vi "deserialize (HW-Ballard).vi"(11 "data in":string[][](array[string])) -> (3 "hw configuration":T1[](array[typedef]))   [LabVIEW 2020]
uses:
  _controls/ballard1553_hw_map.ctl
  _controls/ballard1553_RT_list.ctl
  <vilib>/Utility/miscctls.llb/LVMapReplaceAction.ctl
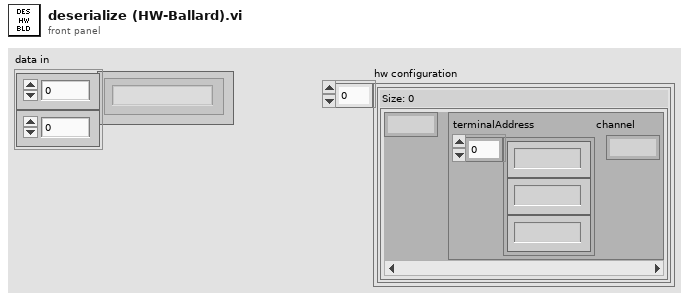
[diagram p1: front panel]
types:
  T1 = typedef "ballard1553_hw_map.ctl" = map{i32, T2}
  T2 = typedef "ballard1553_RT_list.ctl" = cluster{"terminalAddress":i32[], "channel":i32}
  T3 = typedef "LVMapReplaceAction.ctl" = enum32{"Modify Entry only if found", "Add or Modify Entry", "Delete Entry"}
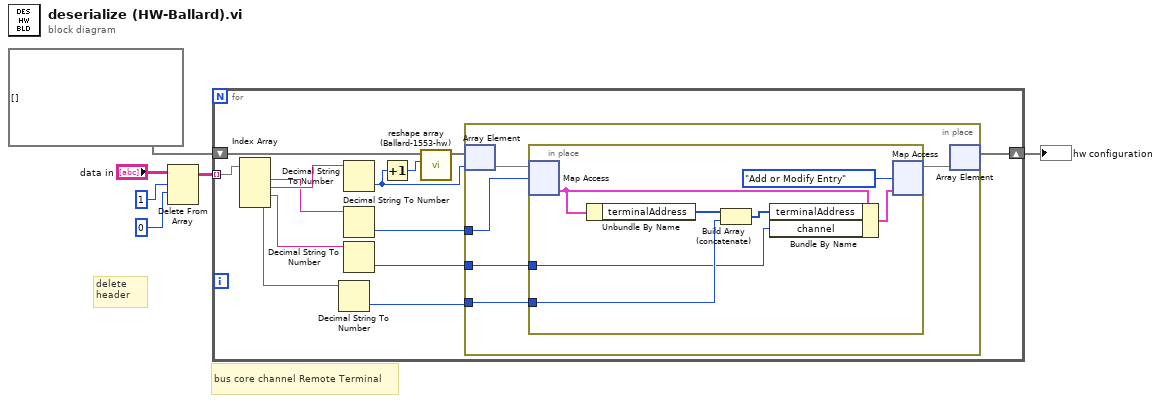
[diagram p0: block diagram]
diagram:
  # "bus\tcore\tchannel\tRemote Terminal"
  # "delete\nheader"
  n1 = Delete From Array(array="data in", length=1, index (row)=0) -> (array with subset deleted=w3:string[][])  [unwired: 1 in, 1 out]
  n2 = for {
    tunnel: w3 -> [w19] mode=indexing
    shift-right: [w17] -> w1
    shift-left: T1[] [] ("hw configuration") -> [w16]
    n3 = Index Array(array=w19) -> (element #1=w11:string, element #2=w12:string, element #3=w10:string, element #4=w8:string)  [unwired: 4 in]
    n4 = Decimal String To Number(string=w8) -> (number=w9:i32)  [unwired: 2 in, 1 out]
    n5 = Decimal String To Number(string=w12) -> (number=w18:i32)  [unwired: 2 in, 1 out]
    n6 = Decimal String To Number(string=w11) -> (number=w7:i32)  [unwired: 2 in, 1 out]
    n7 = Decimal String To Number(string=w10) -> (number=w13:i32)  [unwired: 2 in, 1 out]
    n8 = Increment(x=w18) -> (x+1=w15:i32)
    n9 = call "reshape array (Ballard-1553-hw).vi"("size requested"=w15, "hw configuration in"=w16) -> ("hw configuration out"=w14:T1[])  [unwired: 9 in]
    n10 = in-place {
      in-place-border: w13 -> [w20]
      in-place-border: w9 -> [w21]
      in-place-border: w7 -> [w22]
      n11 = in-place-array #1(w14, w18) -> (w24:T1)
      n12 = in-place {
        in-place-border: w21 -> [w27]
        in-place-border: w20 -> [w25]
        n13 = in-place-map #2(w24, w22) -> (w31:T2)  [unwired: 1 in, 1 out]
        n14 = Unbundle By Name(w31) -> ("terminalAddress"=w28:i32[])
        n15 = Build Array (concatenate)(w28, w27) -> (w26:i32[])
        n16 = Bundle By Name(cluster=w31, "terminalAddress"=w26, "channel"=w25) -> (w30:T2)
        n17 = in-place-map #2(w30, LVMapReplaceAction."Add or Modify Entry" ("action")) -> (w23:T1)  [unwired: 2 out]
      }
      n18 = in-place-array #1(w23) -> (w17:T1[])  [unwired: 1 out]
    }
  }
  "hw configuration" <- w1
